vi "Main.vi"() -> ()   [LabVIEW 2018]
uses:
  Components/VacSys/VacSys.lvclass
panel:
  out "Pressures":dbl[](array[numeric])
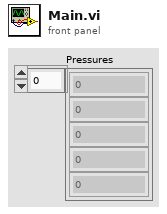
[diagram p1: front panel]
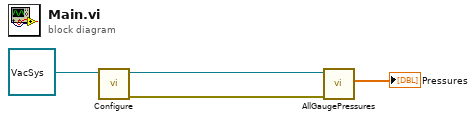
[diagram p0: block diagram]
diagram:
  n1 = call-dynamic "Configure.vi"("VacSys in"=refnum<class "VacSys.lvclass"> refnum ("VacSys.lvclass")) -> ("error out"=w2:errorcluster, "VacSys out"=w3:refnum<class "VacSys.lvclass">)  [unwired: 9 in]
  n2 = call-dynamic "AllGaugePressures.vi"("error in (no error)"=w2, "VacSys in"=w3) -> ("Pressures"=→"Pressures":dbl[])  [unwired: 7 in, 2 out]
